vi "CMI Sync V3 Query.vi"(7 "read byte count (100)":u32=100, 8 "error in":errorcluster, 10 "command":string="*IDN?", 11 "VISA in":refnum<visa-resource-name>) -> (0 "error out":errorcluster, 2 "read buffer":string, 3 "VISA resource name out":refnum<visa-resource-name>)   [LabVIEW 2020, in "AWG.lvlib" / "CMI Sync Unit V3.lvlib"]
doc: "Query answer from sync unit. Automatically appends LF at the end of command, reads till first LF in answer. Flushes read buffer before readout."
uses:
  CMI Sync Unit V3.lvlib
  <vilib>/Instr/_visa.llb/VISA Flush IO Buffer Mask.ctl
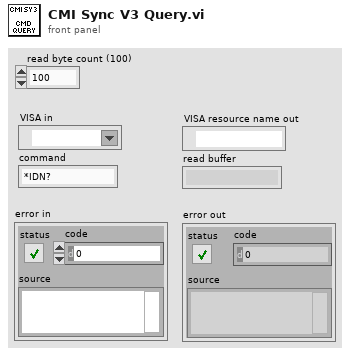
[diagram p1: front panel]
types:
  T1 = typedef "VISA Flush IO Buffer Mask.ctl" = u16
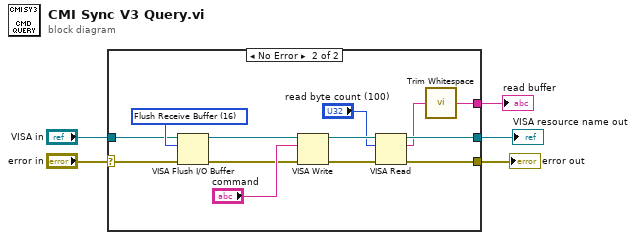
[diagram p0: block diagram]
diagram:
  n1 = case shown="No Error" "error in" {
    selector: "error in" -> [w7 w14]
    tunnel: "VISA in" -> [w6 w19]
    tunnel: [w6 w12] -> w4
    tunnel: [w7 w10] -> w2
    tunnel: [_ w8] -> w1
    frame Error {
    }
    frame No Error {
      w20 = T1 16 items=["Flush Receive Buffer"=16, "Write Transmit Buffer to Device"=32, "Flush Receive Buffer (No I/O)"=64, "Flush Transmit Buffer"=128] ("Mask")
      n2 = VISA Flush I/O Buffer(VISA resource name=w19, mask (16)=w20, error in (no error)=w14) -> (VISA resource name out=w11:refnum<visa-resource-name>, error out=w13:errorcluster)
      n3 = VISA Write(VISA resource name=w11, write buffer="command", error in (no error)=w13) -> (VISA resource name out=w16:refnum<visa-resource-name>, error out=w17:errorcluster)  [unwired: 1 out]
      n4 = VISA Read(VISA resource name=w16, byte count="read byte count (100)", error in (no error)=w17) -> (VISA resource name out=w12:refnum<visa-resource-name>, read buffer=w9:string, error out=w10:errorcluster)  [unwired: 1 out]
      n5 = call <vilib>:"Trim Whitespace.vi"("string"=w9) -> ("trimmed string"=w8:string)  [unwired: 1 in]
    }
  }
  "error out" <- w2
  "VISA resource name out" <- w4
  "read buffer" <- w1
